vi "FetchRemoteLogUI.vi"(10 "Plugin Info":T3, 11 "Remote Logger Input Data":T1) -> ()   [LabVIEW 2016]
uses:
  General/CorePluginInfo.ctl
  LoggerViewerInputData.ctl
  General/RemoteFiles/connectionData.ctl
  LoggerMonitorControlData.ctl
panel:
  out "connectedToLogger":bool caption="Connected to Logger?"
  out "windowName":string
  in  "clearLogBtn":bool
  in  "refreshBtn":bool
  out "Logger Console":string
  in  "viewBtn":bool
  in  "copyBtn":bool
  in  "deleteBtn":bool
  in  "Remote Logs":string(tree)
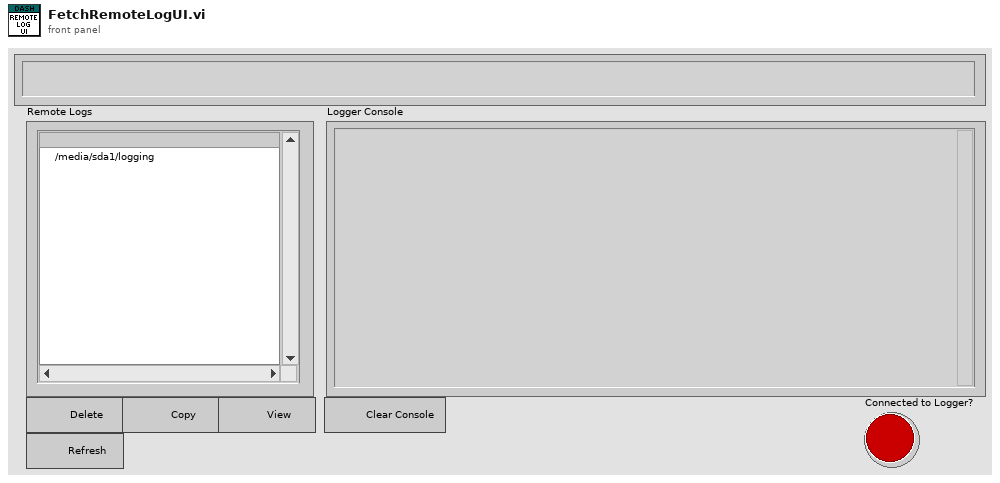
[diagram p1: front panel]
types:
  T1 = typedef "LoggerViewerInputData.ctl" = cluster{"ConnectionData":T2, "BasePath":path, "remotePath":string, "Console buffer size":u32, "remoteLoggerPort":u16}
  T2 = typedef "connectionData.ctl" = cluster{"host":string, "user":string, "password":string, "port":u16}
  T3 = typedef "CorePluginInfo.ctl" = cluster{"Notifiers":cluster{"Robot IP Notifier":refnum<notifier>, "Window Mode Notifier":refnum<notifier>, "Stop Notifier":refnum<notifier>}}
  T4 = typedef "LoggerMonitorControlData.ctl" = cluster{"clearLogBtn":refnum<vi>, "terminalBufferLength(lines)":i32, "remoteLoggerPort":u16, "refreshBtn":refnum<vi>, "Logger Console":refnum<vi>, "ConnectionData":T2, "remotePath":string, "viewBtn":refnum<vi>, "copyBtn":refnum<vi>, "deleteBtn":refnum<vi>, "Remote Logs":refnum<vi>, "windowName":refnum<vi>, "DefaultLocalPath":path, "connectedToLogger":refnum<vi>, "Plugin Info":T3}
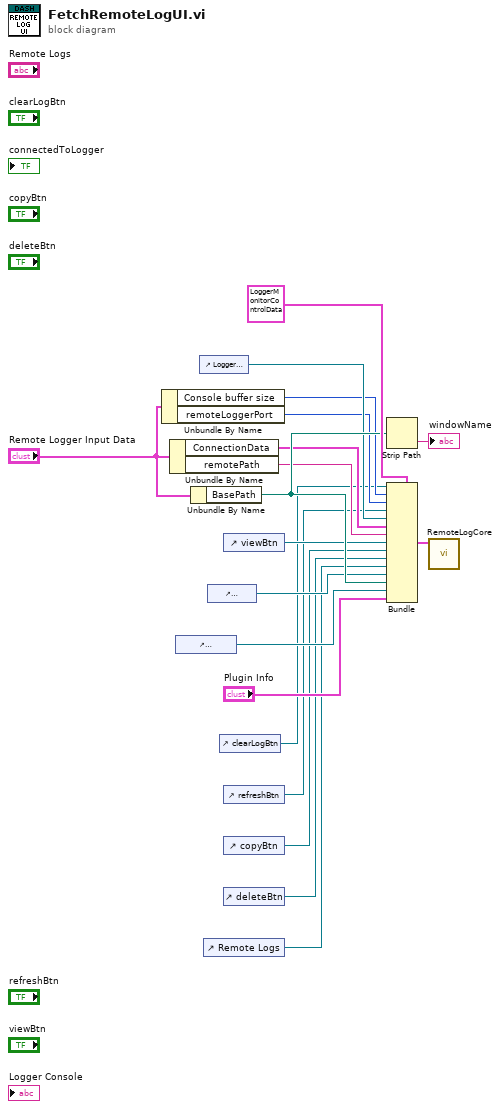
[diagram p0: block diagram]
diagram:
  n1 = Unbundle By Name("Remote Logger Input Data") -> ("Console buffer size"=w3:u32, "remoteLoggerPort"=w2:u16)
  n2 = Unbundle By Name("Remote Logger Input Data") -> ("ConnectionData"=w7:T2, "remotePath"=w8:string)
  n3 = control-ref of="connectedToLogger"() -> (w15:refnum<vi>)
  n4 = Unbundle By Name("Remote Logger Input Data") -> ("BasePath"=w14:path)
  n5 = control-ref of="Logger Console"() -> (w6:refnum<vi>)
  n6 = control-ref of="Remote Logs"() -> (w12:refnum<vi>)
  n7 = control-ref of="windowName"() -> (w13:refnum<vi>)
  n8 = control-ref of="clearLogBtn"() -> (w1:refnum<vi>)
  n9 = control-ref of="viewBtn"() -> (w9:refnum<vi>)
  n10 = control-ref of="refreshBtn"() -> (w5:refnum<vi>)
  n11 = control-ref of="copyBtn"() -> (w10:refnum<vi>)
  n12 = control-ref of="deleteBtn"() -> (w11:refnum<vi>)
  n13 = Strip Path(path=w14) -> (name=→"windowName":string)  [unwired: 1 out]
  n14 = Bundle(cluster=T4 {"clearLogBtn"=refnum, "terminalBufferLength(lines)"=0, "remoteLoggerPort"=0, "refreshBtn"=refnum, "Logger Console"=refnum, "ConnectionData"={"host"="", "user"="", "password"="", "port"=0}, "remotePath"="", "viewBtn"=refnum, "copyBtn"=refnum, "deleteBtn"=refnum, "Remote Logs"=refnum, "windowName"=refnum, "DefaultLocalPath"=path "", "connectedToLogger"=refnum, "Plugin Info"={"Notifiers"={"Robot IP Notifier"=refnum, "Window Mode Notifier"=refnum, "Stop Notifier"=refnum}}} ("LoggerMonitorControlData"), "clearLogBtn"=w1, "terminalBufferLength(lines)"=w3, "remoteLoggerPort"=w2, "refreshBtn"=w5, "Logger Console"=w6, "ConnectionData"=w7, "remotePath"=w8, "viewBtn"=w9, "copyBtn"=w10, "deleteBtn"=w11, "Remote Logs"=w12, "windowName"=w13, "DefaultLocalPath"=w14, "connectedToLogger"=w15, "Plugin Info"="Plugin Info") -> (w18:T4)
  n15 = call "RemoteLogCore.vi"("LoggerMonitorControlData"=w18) -> ()  [unwired: 11 in]
